vi "Write Settings to file.vi"(8 "error in (no error)":errorcluster, 10 "settings":T1, 11 "Configuration Session in":refnum<class "Configuration Session.lvclass">) -> (0 "error out":errorcluster, 2 "settings id":string, 3 "Configuration Session out":refnum<class "Configuration Session.lvclass">)   [LabVIEW 2017, in "DSF Configuration.lvlib" / "Configuration Session.lvclass"]
uses:
  DSF Configuration API/Configuration Session.lvclass
  DSF Configuration API/Public/Controls/DSF Settings Info.ctl
  DSF Configuration API/Public/Write Item/Write Settings.vi
  DSF Configuration.lvlib
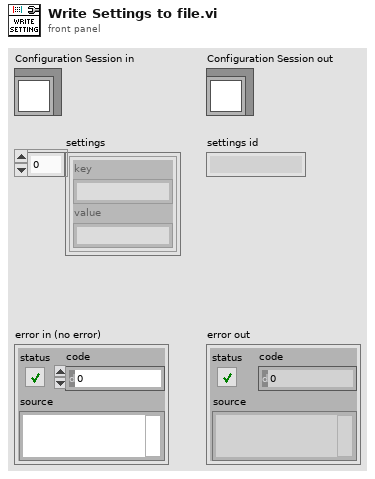
[diagram p1: front panel]
types:
  T1 = typedef "DSF Configuration.lvlib/DSF Settings Info.ctl" = cluster{"key":string, "value":string}[]
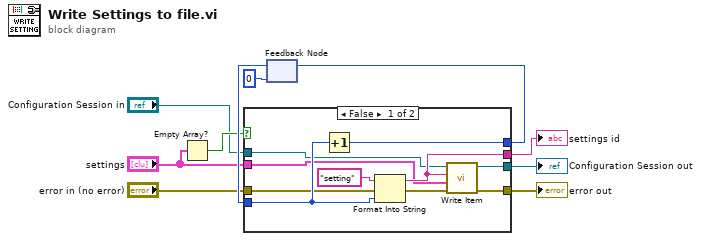
[diagram p0: block diagram]
diagram:
  n1 = Empty Array?(array="settings") -> (empty?=w5:bool)
  n2 = feedback #1(0) -> (w8:i32)
  n3 = case shown="False" w5 {
    tunnel: [w19 w23] -> w9
    tunnel: w8 -> [w18 w23]
    tunnel: [w17 _] -> w10
    tunnel: "settings" -> [w16 _]
    tunnel: "Configuration Session in" -> [w15 w22]
    tunnel: [w14 w22] -> w1
    tunnel: "error in (no error)" -> [w13 w21]
    tunnel: [w11 w21] -> w3
    frame False {
      n4 = Increment(x=w18) -> (x+1=w19:i32)
      n5 = Format Into String(initial string="setting", error in=w13, w18) -> (resulting string=w17:string, error out=w12:errorcluster)  [unwired: 1 in]
      n6 = call-poly "Write Item.vi"("error in (no error)"=w12, "settings values"=w16, "id"=w17, "Configuration Session in"=w15) -> ("error out"=w11:errorcluster, "Configuration Session out"=w14:refnum<class "Configuration Session.lvclass">)  [unwired: 5 in, 1 out]
    }
    frame True {
    }
  }
  "settings id" <- w10
  "error out" <- w3
  "Configuration Session out" <- w1
  n7 = feedback-in #1(w9) -> ()
